vi "PPG_ABC.ProcPeriodic.vi"(0 "i ref in":refnum<vi>, 3 "ms timeout (10000)":i32=10000, 5 "error in (no error)":errorcluster) -> (14 "i ref out":refnum<vi>, 17 "timed out":bool, 19 "error out":errorcluster)   [LabVIEW 2014, in "PPG_ABC.lvlib"]
doc: "This method serves to periodically do things like reading values from the HW. Methods that should be executed periodically should be called from THIS methode. Add code here."
uses:
  PPG_ABC.lvlib
  NI_FPGA_PPG/NI_FPGA_PPG.lvlib
  CSlibraries/UtilityLib/UtilityLib.lvlib
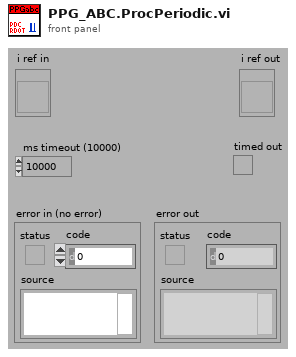
[diagram p1: front panel]
types:
  T1 = typedef "PPG_ABC.lvlib/PPG_ABC.i attribute.ctl" = cluster{"patternGroups":T2[], "defaultLetter":string, "defaultPatternGroup":i32, "PGRunning":T3, "PGRunningID":i32, "pgStarting":T4}
  T2 = typedef "PPG_ABC.lvlib/PPG_ABC.PG_dataType.ctl" = cluster{"PGDevice":string, "rawPatternData":cluster{"triggerCondition":i32, "timeTable":dbl[], "channelTable":string[]}[]}
  T3 = typedef "PPG_ABC.lvlib/PPG_ABC.PG_Running.ctl" = i32
  T4 = typedef "Semaphore RefNum" = refnum<k1>
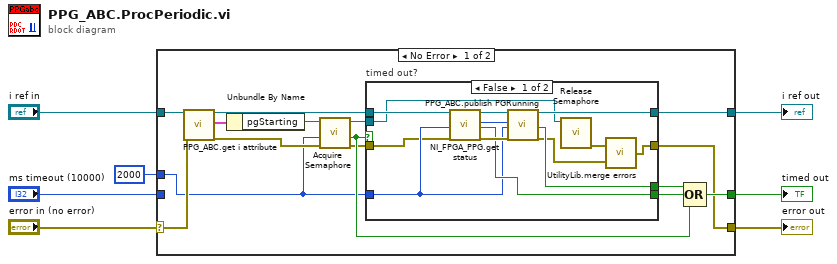
[diagram p0: block diagram]
diagram:
  n1 = case shown="No Error" "error in (no error)" {
    selector: "error in (no error)" -> [w17 w38]
    tunnel: "i ref in" -> [w18 w39]
    tunnel: [w22 w39] -> w6
    tunnel: [w10 w38] -> w5
    tunnel: [w21 _] -> w4
    tunnel: "ms timeout (10000)" -> [_ _]
    tunnel: 2000 ("ms timeout (10000)") -> [w8 _]
    frame No Error {
      n2 = call "PPG_ABC.get i attribute.vi"("i ref in"=w18, "error in (no error)"=w17) -> ("i ref out"=w13:refnum<vi>, "i attribute"=w16:T1, "error out"=w14:errorcluster)  [unwired: 15 in]
      n3 = Unbundle By Name(w16) -> ("pgStarting"=w15:T4)
      n4 = call <vilib>:"Acquire Semaphore.vi"("error in (no error)"=w14, "ms timeout (-1)"=w8, "semaphore"=w15) -> ("error out"=w11:errorcluster, "timed out"=w12:bool, "semaphore out"=w9:T4)  [unwired: 2 in]
      n5 = case "timed out?" shown="False" w12 {
        tunnel: [w33 w37] -> w22
        tunnel: [w32 _] -> w20
        tunnel: [w30 _] -> w19
        tunnel: w8 -> [w29 _]
        tunnel: w13 -> [w27 w37]
        tunnel: w11 -> [w28 w36]
        tunnel: [w24 w36] -> w10
        tunnel: w9 -> [w26 _]
        frame False {
          n6 = call "NI_FPGA_PPG.get status.vi"("i ref in"=w27, "ms timeout (10000)"=w29, "error in (no error)"=w28) -> ("i ref out"=w35:refnum<vi>, "FPGA_status"=w31:i32, "timed out"=w30:bool, "error out"=w34:errorcluster)  [unwired: 13 in]
          n7 = call "PPG_ABC.publish PGRunning.vi"("i ref in"=w35, "PPGRunning"=w31, "ms timeout (10000)"=w29, "error in (no error)"=w34) -> ("i ref out"=w33:refnum<vi>, "timed out"=w32:bool, "error out"=w23:errorcluster)  [unwired: 13 in]
          n8 = call <vilib>:"Release Semaphore.vi"("semaphore"=w26) -> ("error out"=w25:errorcluster)  [unwired: 5 in, 1 out]
          n9 = call "UtilityLib.merge errors.vi"("error2 (no error)"=w23, "error1 (no error)"=w25) -> ("error out"=w24:errorcluster)
        }
        frame True {
        }
      }
      n10 = Compound Arithmetic op=OR(w20, w19, w12) -> (w21:bool)
    }
    frame Error {
    }
  }
  "error out" <- w5
  "i ref out" <- w6
  "timed out" <- w4
